vi "DSF.Engine.Runtime.Framework.Get Sequencer.vi"(8 "error in (no error)":errorcluster, 11 "Framework Runtime in":refnum<class "DSF.Engine.Runtime.Framework.lvclass">) -> (0 "error out":errorcluster, 2 "Sequencer":refnum<class "DSF.Engine.Sequencer.lvclass">, 3 "Framework Runtime out":refnum<class "DSF.Engine.Runtime.Framework.lvclass">)   [LabVIEW 2017, in "DSF.Engine.lvlib" / "DSF.Engine.Runtime.Framework.lvclass"]
uses:
  DSF.Engine.Runtime.Framework.lvclass
  Sequencer/DSF.Engine.Sequencer.lvclass
  DSF.Engine.Runtime.Framework.lvclass/DSF.Engine.Runtime.Framework.ctl
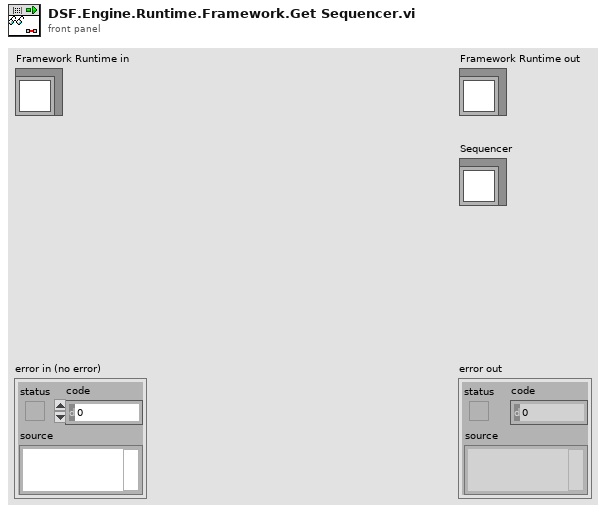
[diagram p1: front panel]
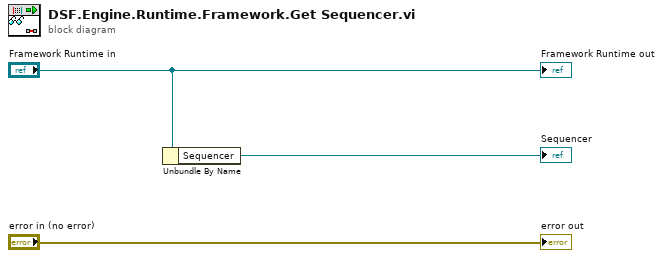
[diagram p0: block diagram]
diagram:
  n1 = Unbundle By Name("Framework Runtime in") -> ("Sequencer"=→"Sequencer":refnum<class "DSF.Engine.Sequencer.lvclass">)
  "error out" <- "error in (no error)"
  "Framework Runtime out" <- "Framework Runtime in"
